vi "fgv_ctrl-ref2.vi"(7 "cmd":T2, 11 "input cluster":T1) -> (3 "input cluster 2":T1)   [LabVIEW 2019]
uses:
  ref.ctl
  _ctrl/rw.ctl
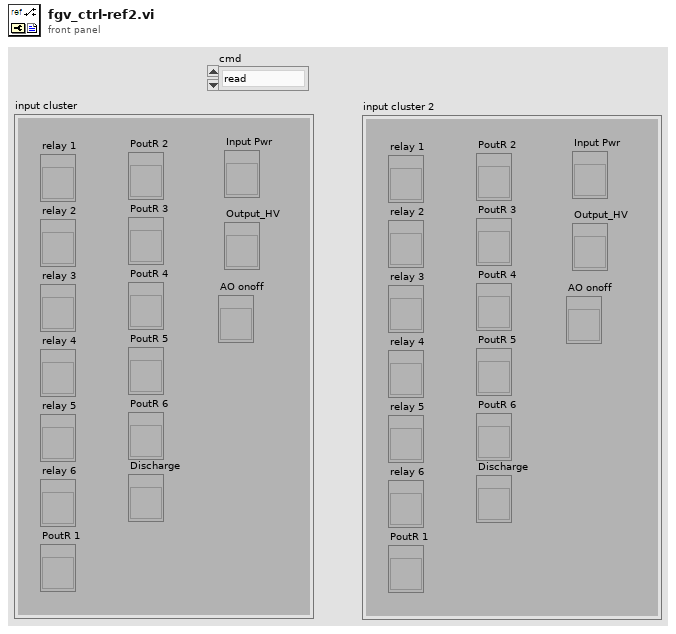
[diagram p1: front panel]
types:
  T1 = typedef "ref.ctl" = cluster{"relay 1":refnum<vi>, "relay 2":refnum<vi>, "relay 3":refnum<vi>, "relay 4":refnum<vi>, "relay 5":refnum<vi>, "relay 6":refnum<vi>, "PoutR 1":refnum<vi>, "PoutR 2":refnum<vi>, "PoutR 3":refnum<vi>, "PoutR 4":refnum<vi>, "PoutR 5":refnum<vi>, "PoutR 6":refnum<vi>, "Discharge":refnum<vi>, "Input Pwr":refnum<vi>, "Output_HV":refnum<vi>, "AO onoff":refnum<vi>}
  T2 = typedef "rw.ctl" = enum16{"read", "write"}
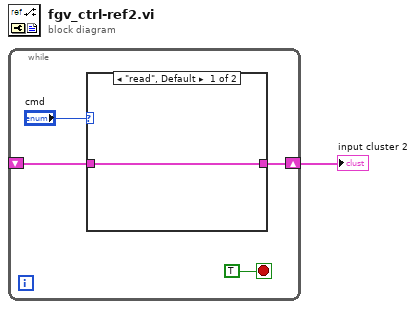
[diagram p0: block diagram]
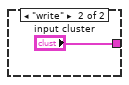
[diagram p2: hidden frame]
diagram:
  n1 = while {
    shift-right: [w3] -> w1
    shift-left: _ -> [w2]
    stop <- TRUE stop-if-true
    n2 = case shown="\"read\", Default" "cmd" {
      tunnel: [w6 "input cluster"] -> w3
      tunnel: w2 -> [w6 _]
      frame "read", Default {
      }
      frame "write" {
      }
    }
  }
  "input cluster 2" <- w1
